vi "Write Timing.vi"(8 "error in (no error)":errorcluster, 10 "Timing":T1={"Sampling"={"Fs"=1000.0, "#s"=128}, "Fs_Out"=10123.0} {"Sampling"."Fs" format="%#_13g"}, 11 "DSP in":refnum<class "DSP.lvclass">) -> (0 "error out":errorcluster, 3 "DSP out":refnum<class "DSP.lvclass">)   [LabVIEW 2019, in "DSP.lvclass"]
uses:
  DSP.lvclass
  Typedefs/DSP.Config.Timing--Cluster.ctl
  DSP.lvclass/DSP.ctl
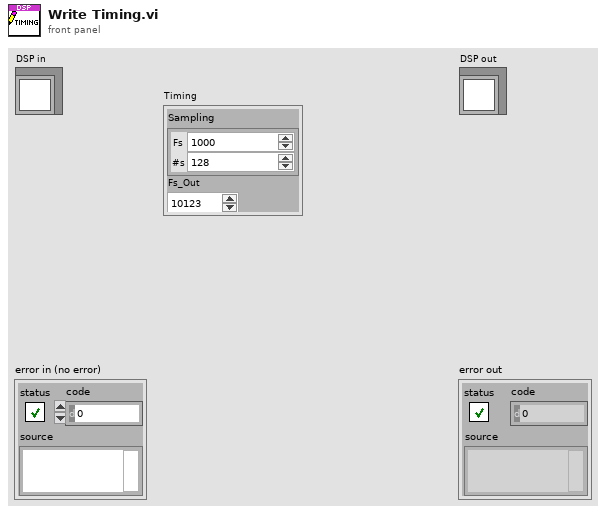
[diagram p1: front panel]
types:
  T1 = typedef "DSP.lvclass/DSP.Config.Timing--Cluster.ctl" = cluster{"Sampling":cluster{"Fs":dbl, "#s":i32}, "Fs_Out":dbl}
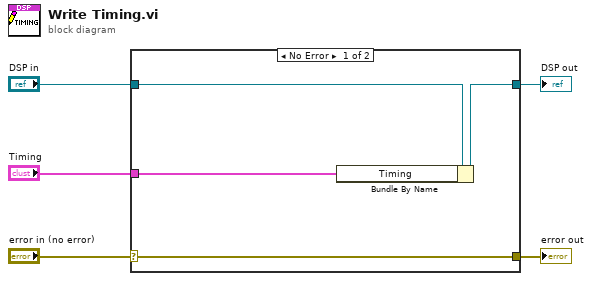
[diagram p0: block diagram]
diagram:
  n1 = case shown="No Error" "error in (no error)" {
    selector: "error in (no error)" -> [w9 w10]
    tunnel: [w9 w10] -> w4
    tunnel: [w7 w11] -> w2
    tunnel: "DSP in" -> [w8 w11]
    tunnel: "Timing" -> [w6 _]
    frame No Error {
      n2 = Bundle By Name(cluster=w8, "Timing"=w6) -> (w7:refnum<class "DSP.lvclass">)
    }
    frame Error {
    }
  }
  "error out" <- w4
  "DSP out" <- w2
